vi "append1DColumn--boolean.vi"(6 "Style":refnum<class "Style.lvclass">, 8 "error in (no error)":errorcluster, 10 "Value":bool[](array[boolean]), 11 "MS-Excel in":refnum<class "MS-Excel.lvclass">) -> (0 "error out":errorcluster, 3 "MS-Excel out":refnum<class "MS-Excel.lvclass">)   [LabVIEW 2017, in "LabVIEW NPOI.lvlib" / "MS-Excel.lvclass"]
uses:
  MS-Excel.lvclass
  D:/Benjamin/Documents/Perso/Code/WC/LabVIEW_NPOI/lib/NPOI 2.1.1/NPOI.dll
  lib/NPOI 2.1.1/NPOI.dll
  Styles/Style/Style.lvclass
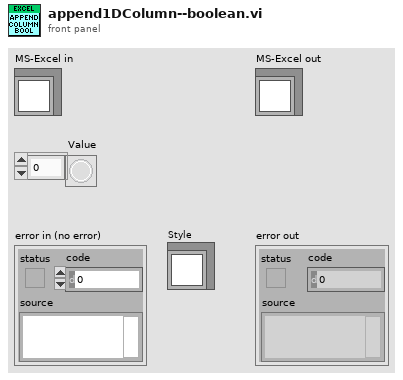
[diagram p1: front panel]
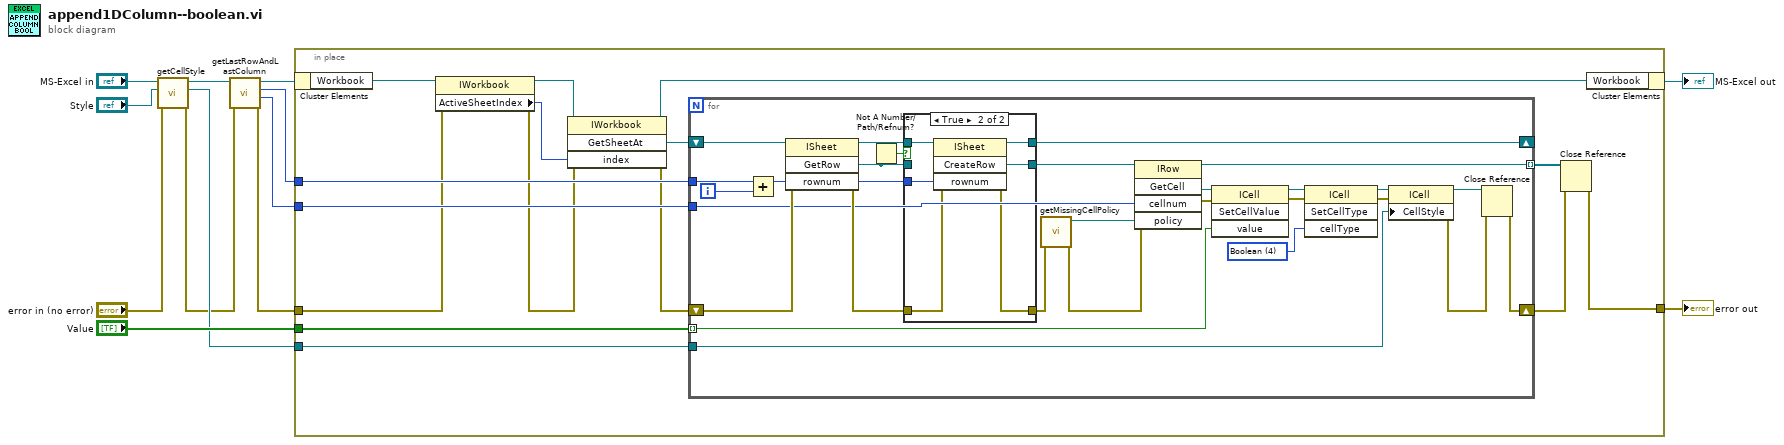
[diagram p0: block diagram]
diagram:
  n1 = call-dynamic "getCellStyle.vi"("error in (no error)"="error in (no error)", "Style"="Style", "MS-Excel in"="MS-Excel in") -> ("error out"=w1:errorcluster, "Cell Style"=w3:refnum<k24>, "MS-Excel out"=w5:refnum<class "MS-Excel.lvclass">)  [unwired: 6 in]
  n2 = call-dynamic "getLastRowAndLastColumn.vi"("error in (no error)"=w1, "MS-Excel in"=w5) -> ("error out"=w8:errorcluster, "Last Column"=w6:i32, "Last Row"=w7:i32, "MS-Excel out"=w9:refnum<class "MS-Excel.lvclass">)  [unwired: 6 in]
  n3 = in-place {
    in-place-border: w8 -> [w17]
    in-place-border: [w23] -> w12
    in-place-border: w7 -> [w28]
    in-place-border: w6 -> [w27]
    in-place-border: "Value" -> [w26]
    in-place-border: w3 -> [w14]
    n4 = in-place-cluster #1(w9) -> ("Workbook"=w15:refnum<k24>)
    n5 = property class="IWorkbook"(reference=w15, error in=w17) -> (reference out=w19:refnum<k24>, error out=w16:errorcluster, "ActiveSheetIndex"=w18:i32)
    n6 = invoke class="IWorkbook" method="GetSheetAt"(reference=w19, error in=w16, "index"=w18) -> (reference out=w21:refnum<k24>, error out=w20:errorcluster, "GetSheetAt"=w22:refnum<k24>)  [unwired: 1 in, 1 out]
    n7 = for {
      tunnel: w28 -> [w52]
      shift-right: [w51] -> _
      shift-left: w22 -> [w56]
      shift-right: [w43] -> w24
      shift-left: w20 -> [w49]
      tunnel: w27 -> [w29]
      tunnel: w26 -> [w46] mode=indexing
      tunnel: [w42] -> w25 mode=indexing
      tunnel: w14 -> [w37]
      i -> [w41]
      w32 = 4 items=["Numeric"=0, "String"=1, "Formula"=2, "Blank"=3, "Boolean"=4, "Error"=5, "Unknown"=-1] ("cellType")
      n8 = Add(x=w52, y=w41) -> (x+y=w47:i32)
      n9 = invoke class="ISheet" method="GetRow"(reference=w56, error in=w49, "rownum"=w47) -> (reference out=w53:refnum<k24>, error out=w50:errorcluster, "GetRow"=w54:refnum<k24>)  [unwired: 1 in, 1 out]
      n10 = Not A Number/Path/Refnum?(number/path/refnum=w54) -> (NaN/Path/Refnum?=w55:bool)
      n11 = case shown="True" w55 {
        tunnel: w54 -> [w58 _]
        tunnel: w53 -> [w57 w65]
        tunnel: w47 -> [_ w64]
        tunnel: w50 -> [w59 w60]
        tunnel: [w59 w62] -> w39
        tunnel: [w58 w63] -> w48
        tunnel: [w57 w61] -> w51
        frame False {
        }
        frame True {
          n12 = invoke class="ISheet" method="CreateRow"(reference=w65, error in=w60, "rownum"=w64) -> (reference out=w61:refnum<k24>, error out=w62:errorcluster, "CreateRow"=w63:refnum<k24>)  [unwired: 1 in, 1 out]
        }
      }
      n13 = call "getMissingCellPolicy.vi"("error in (no error)"=w39) -> ("error out"=w38:errorcluster, "CREATE_NULL_AS_BLANK"=w40:refnum<k24>)  [unwired: 9 in]
      n14 = invoke class="IRow" method="GetCell"(reference=w48, error in=w38, "cellnum"=w29, "policy"=w40) -> (reference out=w42:refnum<k24>, error out=w35:errorcluster, "GetCell"=w36:refnum<k24>)  [unwired: 1 in, 2 out]
      n15 = invoke class="ICell" method="SetCellValue"(reference=w36, error in=w35, "value"=w46) -> (reference out=w34:refnum<k24>, error out=w33:errorcluster)  [unwired: 1 in, 2 out]
      n16 = invoke class="ICell" method="SetCellType"(reference=w34, error in=w33, "cellType"=w32) -> (reference out=w31:refnum<k24>, error out=w30:errorcluster)  [unwired: 1 in, 2 out]
      n17 = property class="ICell"(reference=w31, error in=w30, "CellStyle"=w37) -> (reference out=w45:refnum<k24>, error out=w44:errorcluster)
      n18 = Close Reference(reference=w45, error in (no error)=w44) -> (error out=w43:errorcluster)
    }
    n19 = Close Reference(reference=w25, error in (no error)=w24) -> (error out=w23:errorcluster)
    n20 = in-place-cluster #1("Workbook"=w21) -> (→"MS-Excel out":refnum<class "MS-Excel.lvclass">)
  }
  "error out" <- w12
